vi "clear Session Data.vi"(0 "OBJ - Measurement Session in":refnum<class "File Session.lvclass">, 11 "error in":errorcluster) -> (4 "OBJ - Measurement Session out":refnum<class "File Session.lvclass">, 15 "error out":errorcluster)   [LabVIEW 2015, in "File Session.lvclass"]
doc: "OVERRIDE VI\nPlaceholder for decendant classes to clear session information and close references."
uses:
  File Session.lvclass
  File Session.lvclass/File Session.ctl
  Accessors/Read FileRef.vi
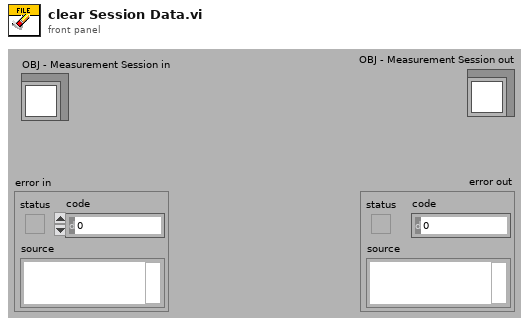
[diagram p1: front panel]
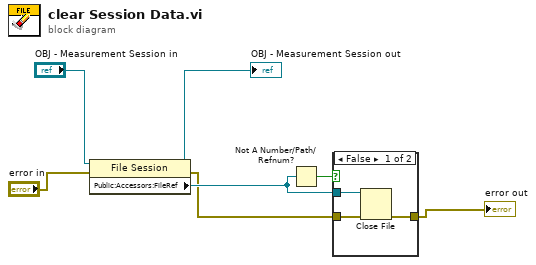
[diagram p0: block diagram]
diagram:
  n1 = property class="File Session"(reference="OBJ - Measurement Session in", error in="error in") -> (reference out=→"OBJ - Measurement Session out":refnum<class "File Session.lvclass">, error out=w4:errorcluster, "Public:Accessors:FileRef"=w5:refnum<file>)
  n2 = Not A Number/Path/Refnum?(number/path/refnum=w5) -> (NaN/Path/Refnum?=w7:bool)
  n3 = case shown="False" w7 {
    tunnel: w4 -> [w10 w11]
    tunnel: [w9 w11] -> w2
    tunnel: w5 -> [w8 _]
    frame False {
      n4 = Close File(refnum=w8, error in=w10) -> (error out=w9:errorcluster)  [unwired: 1 out]
    }
    frame True {
    }
  }
  "error out" <- w2
